vi "Cluster_1.vi"() -> ()   [LabVIEW 2016]
panel:
  in  "Cluster":T1
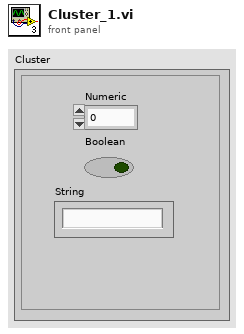
[diagram p1: front panel]
types:
  T1 = cluster{"Numeric":dbl, "Boolean":bool, "String":string}
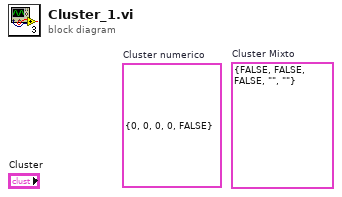
[diagram p0: block diagram]
diagram:
  (unwired) cluster{bool, bool, bool, string, string} {FALSE, FALSE, FALSE, "", ""}  # Cluster Mixto
  (unwired) cluster{i32, i32, i32, i32, bool} {0, 0, 0, 0, FALSE}  # Cluster numerico
